vi "Generate Unique Header.vi"(8 "error in":errorcluster, 11 "Alicat Data in":refnum<class "Alicat Data.lvclass">) -> (0 "error out":errorcluster, 2 "Header":string[](array[string]), 3 "Alicat Data out":refnum<class "Alicat Data.lvclass">)   [LabVIEW 2014, in "Alicat Lib.lvlib" / "Alicat Data.lvclass"]
uses:
  Alicat Data.lvclass
  reusable/Data/Data.lvclass/Data.ctl
  reusable/Data/Read Data ID.vi
  reusable/Data/Data.lvclass
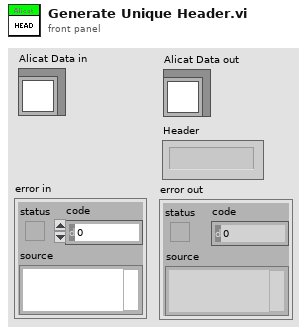
[diagram p1: front panel]
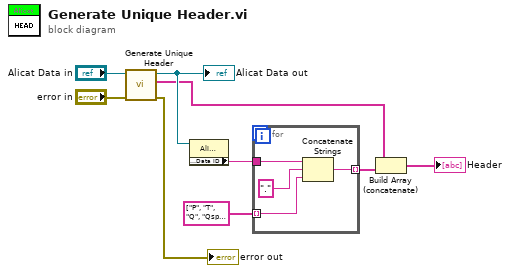
[diagram p0: block diagram]
diagram:
  n1 = call-parent "Generate Unique Header.vi"("error in"="error in", "Data in"="Alicat Data in") -> ("error out"=→"error out":errorcluster, "Header"=w2:string[], "Data out"=w5:refnum<class "Alicat Data.lvclass">)  [unwired: 7 in]
  "Alicat Data out" <- w5
  n2 = property class="Alicat Data"(reference=w5) -> ("Accessors:Data ID"=w4:string)  [unwired: 1 in, 2 out]
  n3 = for {
    tunnel: string[] ["P", "T", "Q", "Qsp", "Q0"] -> [w10] mode=indexing
    tunnel: w4 -> [w13]
    tunnel: [w12] -> w3 mode=indexing
    n4 = Concatenate Strings(w13, "." ("string"), w10) -> (w12:string)
  }
  n5 = Build Array (concatenate)(w2, w3) -> (→"Header":string[])
